vi "add pair to buddle.vi"(5 "y":dbl, 7 "x":dbl, 11 "Input":cluster{dbl[], dbl[]}) -> (3 "output":cluster{dbl[], dbl[]})   [LabVIEW 2024]
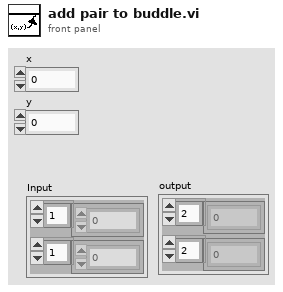
[diagram p1: front panel]
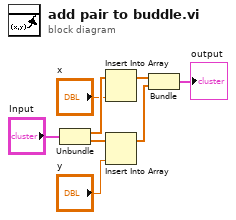
[diagram p0: block diagram]
diagram:
  n1 = Unbundle("Input") -> (w7:dbl[], w5:dbl[])
  n2 = Insert Into Array(array=w7, new element="x") -> (w3:dbl[])  [unwired: 1 in]
  n3 = Insert Into Array(array=w5, new element="y") -> (w2:dbl[])  [unwired: 1 in]
  n4 = Bundle(w3, w2) -> (→"output":cluster{dbl[], dbl[]})  [unwired: 1 in]
